vi "console_journal.vi"(8 "entrée d'erreur (pas d'erreur)":errorcluster) -> (0 "sortie d'erreur":errorcluster)   [LabVIEW 2020]
uses:
  Modules/FS/60_FS_Controles/60_FS_SetGet.ctl
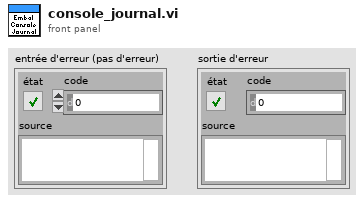
[diagram p1: front panel]
types:
  T1 = typedef "60_FS_SetGet.ctl" = enum16{"set", "get"}
  T2 = typedef "60_FS_CLT_Chemins.ctl" = cluster{"Racine_local":path, "Racine_reseau":path, "Racine_Support_Application":path, "Fichier_Journalisation":path, "Connexion_BDD_VSX":path, "Connexion_BDD_PLZ":path}
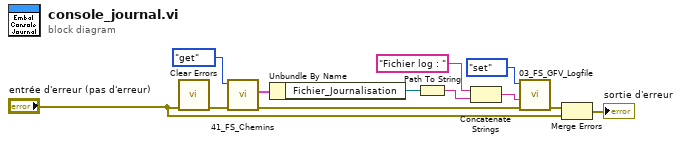
[diagram p0: block diagram]
diagram:
  n1 = call <vilib>:"Clear Errors.vi"("error in (no error)"="entrée d'erreur (pas d'erreur)") -> ("error out"=w3:errorcluster)  [unwired: 5 in, 1 out]
  n2 = call "41_FS_Chemins.vi"("error in (no error)"=w3, "SetGet"=60_FS_SetGet."get") -> ("error out"=w11:errorcluster, "CLT_Chemins_out"=w6:T2)  [unwired: 8 in]
  n3 = Unbundle By Name(w6) -> ("Fichier_Journalisation"=w9:path)
  n4 = Path To String(path=w9) -> (string=w12:string)
  n5 = Concatenate Strings("Fichier log : " ("chaîne"), w12) -> (w8:string)
  n6 = call "03_FS_GFV_Logfile.vi"("error in"=w11, "Chaîne"=w8, "States"=60_FS_SetGet."set") -> ("error out"=w1:errorcluster)  [unwired: 7 in, 1 out]
  n7 = Merge Errors(w1, "entrée d'erreur (pas d'erreur)") -> (→"sortie d'erreur":errorcluster)
